vi "test - read value with backslash.vi"(8 "error in (no error)":errorcluster, 11 "TestCase in":refnum<class "csm-ini-variable-addon.lvclass">) -> (0 "error out":errorcluster, 3 "TestCase out":refnum<class "csm-ini-variable-addon.lvclass">)   [LabVIEW 2017, in "csm-ini-variable-addon.lvclass"]
uses:
  csm-ini-variable-addon.lvclass
  <vilib>/addons/_JKI Toolkits/VI Tester/TestCase.llb/TestCase.lvclass
  INI-Static-Variable-Support/INI-Static-Variable-Support.lvlib
  <userlib>/_NEVSTOP/Communicable State Machine(CSM)/addons/API-String-Arugments-Support/API String Arguments Support.lvlib
  C:/Program Files (x86)/National Instruments/LabVIEW 2017/vi.lib/addons/_JKI Toolkits/VI Tester/TestCase.llb/TestCase.lvclass
panel:
  out "String out":string
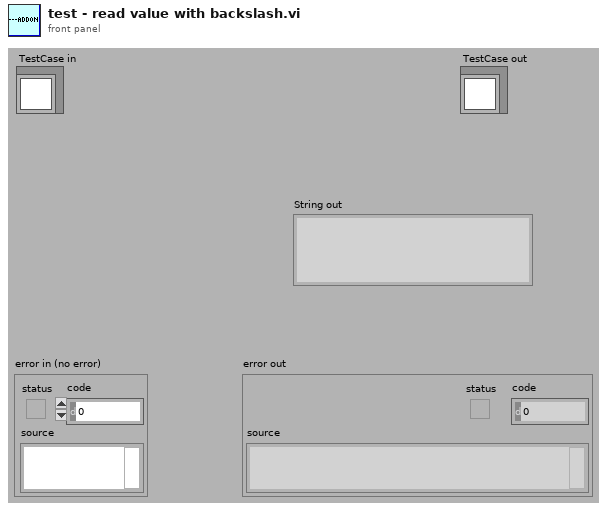
[diagram p1: front panel]
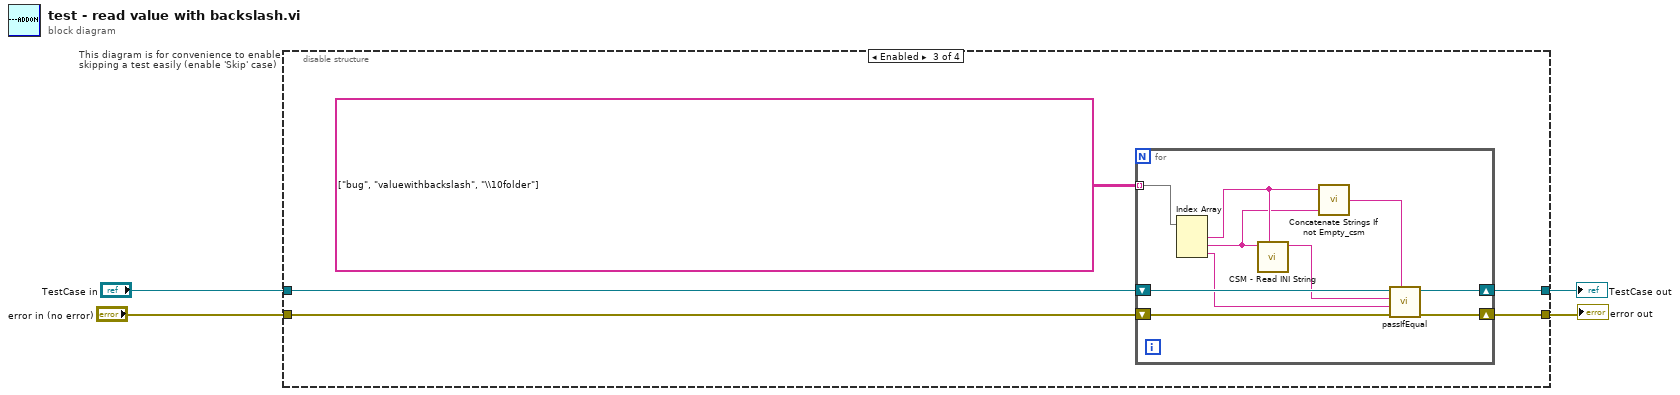
[diagram p0: block diagram]
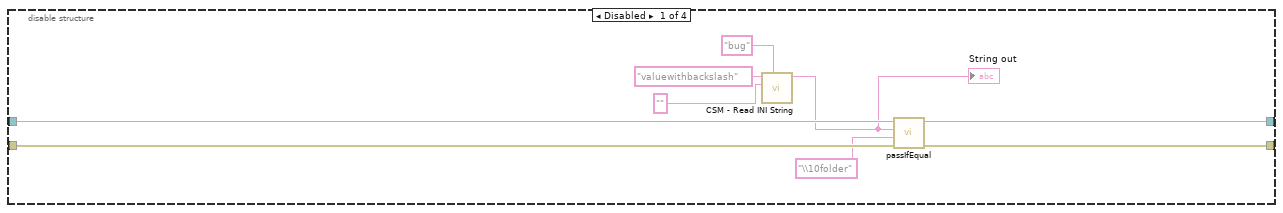
[diagram p2: hidden frame]
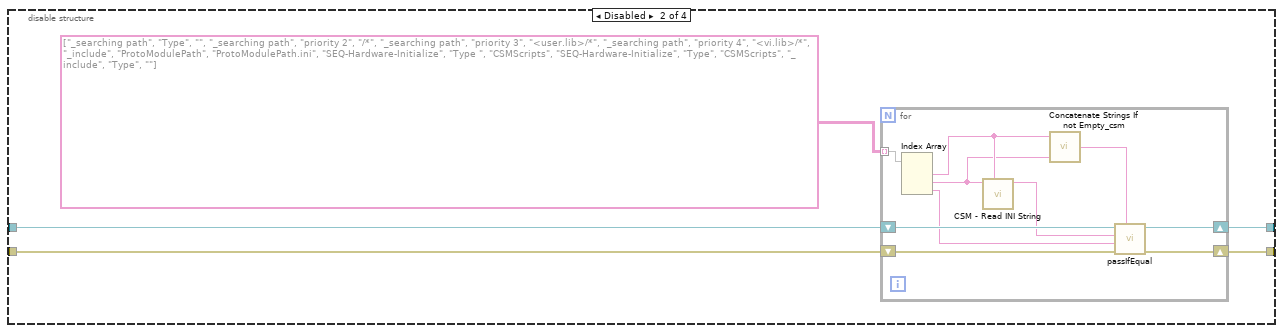
[diagram p3: hidden frame]
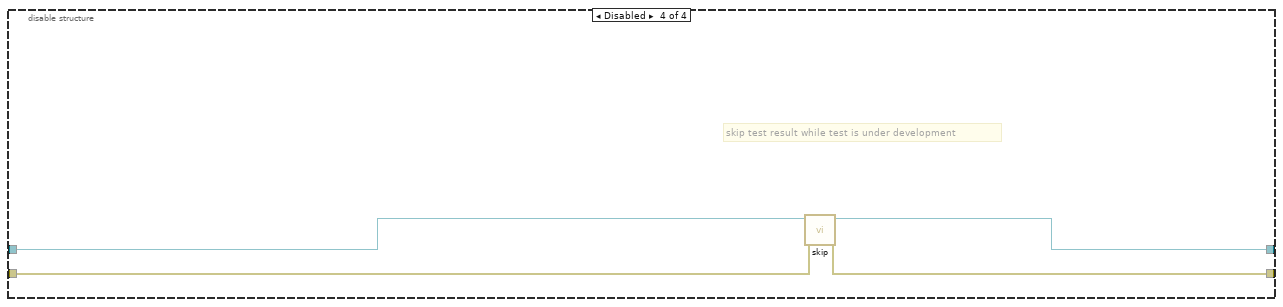
[diagram p4: hidden frame]
diagram:
  n1 = disable-structure "This diagram is for convenience to enable skipping a test easily (enable 'Skip' case)" shown="Enabled" {
    disable-tunnel: "TestCase in" -> [w10 w15 w30 w47]
    disable-tunnel: [w13 w18 w33 w45] -> w1
    disable-tunnel: [w12 w17 w32 w46] -> w3
    disable-tunnel: "error in (no error)" -> [w11 w16 w31 w44]
    frame Disabled {
      n2 = call "CSM - Read INI String.vi"("Section Name(\"\" as Default)"="bug" ("Section Name(\"\" as Default)"), ">> Default Value >>"="" ("String in"), "String in"="valuewithbackslash") -> ("String out"=w6:string)  [unwired: 4 in, 2 out]
      "String out" <- w6
      n3 = call-dynamic "passIfEqual.vi"("error in (no error)"=w11, "y"="\\10folder" ("String in"), "x"=w6, "TestCase in"=w10) -> ("error out"=w12:errorcluster, "TestCase out"=w13:refnum<class "csm-ini-variable-addon.lvclass">)  [unwired: 6 in]
    }
    frame Disabled {
      n4 = for {
        shift-right: [w27] -> w17
        shift-left: w16 -> [w26]
        shift-right: [w28] -> w18
        shift-left: w15 -> [w25]
        tunnel: string[][] [["_searching path", "Type", ""], ["_searching path", "priority 2", "/*"], ["_searching path", "priority 3", "<user.lib>/*"], ["_searching path", "priority 4", "<vi.lib>/*"], ["_include", "ProtoModulePath", "ProtoModulePath.ini"], ["SEQ-Hardware-Initialize", "Type ", "CSMScripts"], ["SEQ-Hardware-Initialize", "Type", "CSMScripts"], ["_include", "Type", ""]] -> [w23] mode=indexing
        n5 = Index Array(array=w23) -> (element #1=w20:string, element #2=w19:string, element #3=w22:string)  [unwired: 3 in]
        n6 = call "CSM - Read INI String.vi"("Section Name(\"\" as Default)"=w20, "String in"=w19) -> ("String out"=w24:string)  [unwired: 5 in, 2 out]
        n7 = call <userlib>:"Concatenate Strings If not Empty_csm.vi"("String"=w19, "prefix"=w20) -> ("result"=w21:string)  [unwired: 3 in]
        n8 = call-dynamic "passIfEqual.vi"("custom report message (\"\")"=w21, "error in (no error)"=w26, "y"=w22, "x"=w24, "TestCase in"=w25) -> ("error out"=w27:errorcluster, "TestCase out"=w28:refnum<class "csm-ini-variable-addon.lvclass">)  [unwired: 5 in]
      }
    }
    frame Enabled {
      n9 = for {
        shift-right: [w42] -> w32
        shift-left: w31 -> [w41]
        shift-right: [w43] -> w33
        shift-left: w30 -> [w40]
        tunnel: string[][] [["bug", "valuewithbackslash", "\\10folder"]] -> [w38] mode=indexing
        n10 = Index Array(array=w38) -> (element #1=w35:string, element #2=w34:string, element #3=w37:string)  [unwired: 3 in]
        n11 = call "CSM - Read INI String.vi"("Section Name(\"\" as Default)"=w35, "String in"=w34) -> ("String out"=w39:string)  [unwired: 5 in, 2 out]
        n12 = call <userlib>:"Concatenate Strings If not Empty_csm.vi"("String"=w34, "prefix"=w35) -> ("result"=w36:string)  [unwired: 3 in]
        n13 = call-dynamic "passIfEqual.vi"("custom report message (\"\")"=w36, "error in (no error)"=w41, "y"=w37, "x"=w39, "TestCase in"=w40) -> ("error out"=w42:errorcluster, "TestCase out"=w43:refnum<class "csm-ini-variable-addon.lvclass">)  [unwired: 5 in]
      }
    }
    frame Disabled {
      # "skip test result while test is under development"
      n14 = call <vilib>:"skip.vi"("error in (no error)"=w44, "TestCase in"=w47) -> ("error out"=w46:errorcluster, "TestCase out"=w45:refnum<class "csm-ini-variable-addon.lvclass">)  [unwired: 8 in]
    }
  }
  "error out" <- w3
  "TestCase out" <- w1
